vi "Modes_abbrev_global.vi"() -> ()   [LabVIEW 2017, in "XDataNode.xnode"]
uses:
  <vilib>/Platform/TimedLoop/XDataNode/XDataNode.xnode
panel:
  in  "Displayed Abbreviations":string[](array[string])=["NC", "P,M", "D,M", "P,I", "D,I"]
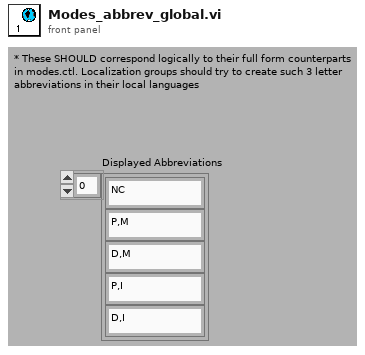
[diagram p1: front panel]
diagram:
